vi "TimedLoop-all-inputs-wired.vi"() -> ()   [LabVIEW 2026]
doc: "This VI illustrates how to use the Stop Timed Structure VI to programmatically abort a Timed Loop."
uses:
  <vilib>/Platform/TimedLoop/XDataNode/timing_clust.ctl
  <vilib>/Platform/TimedLoop/XDataNode/nitl_modes.ctl
  <vilib>/Platform/TimedLoop/XDataNode/wakeup.ctl
  <vilib>/platform/TimedLoop/XDataNode/XDataNode.xnode
  <vilib>/Platform/TimedLoop/XDataNode/XDNodeRunTimeDep.lvlib
panel:
  out "Wakeup Reason":string
  in  "Abort Message":string="The Timed Loop was aborted."
  in  "Abort":bool
  out "Current Iteration":i32
  # "Overview: Demonstrates the use of the Stop Timed Structure VI to programmatically abort a Timed Loop.\nRequirements: Windows\nInstructions:\n1. Run the VI.\n2. Click the Abort Timed Loop button. A dialog will indicate that the Timed Loop was programmatically aborted."
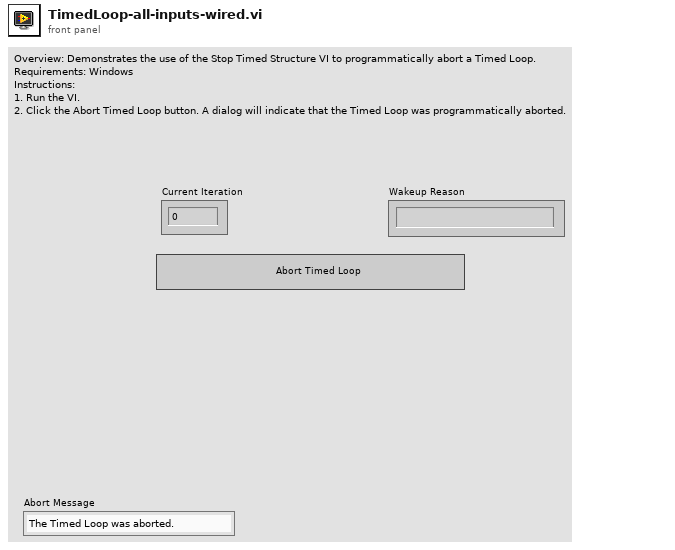
[diagram p1: front panel]
types:
  T1 = typedef "XDNodeRunTimeDep.lvlib/nitl_modes.ctl" = enum32{"No Change", "Process missed periods, maintain original phase", "Discard missed periods, maintain original phase", "Process missed periods, ignore original phase", "Discard missed periods, ignore original phase"}
  T2 = typedef "XDNodeRunTimeDep.lvlib/timing_clust.ctl" = cluster{"Expected End [f-1]":u64, "Actual End [f-1]":u64, "Finished Late? [f-1]":bool, "Expected End [i-1]":u64, "Actual End [i-1]":u64, "Finished Late? [i-1]":bool, "Expected Start [i]":u64, "Actual Start [i]":u64, "Expected Start [f]":u64, "Actual Start [f]":u64, "Source Name":string, "Structure Name":string, "Period":i64, "Deadline":i64, "Offset":i64, "Start":i64, "Priority":i32, "Timeout":i32, "Mode":T1, "Wakeup Reason":T3, "Error":errorcluster, "Source Type":string, "Secondary Source Type":string, "Global End Time":u64, "Global Start Time":u64, "Frame Duration":u64, "Iteration Duration":u64, "Assigned CPU":i32, "I/O Scan Engine Mode":u32}
  T3 = typedef "XDNodeRunTimeDep.lvlib/wakeup.ctl" = enum32{"Normal", "Aborted", "Asynchronous wakeup", "Timing source error", "Timed loop error", "Timeout"}
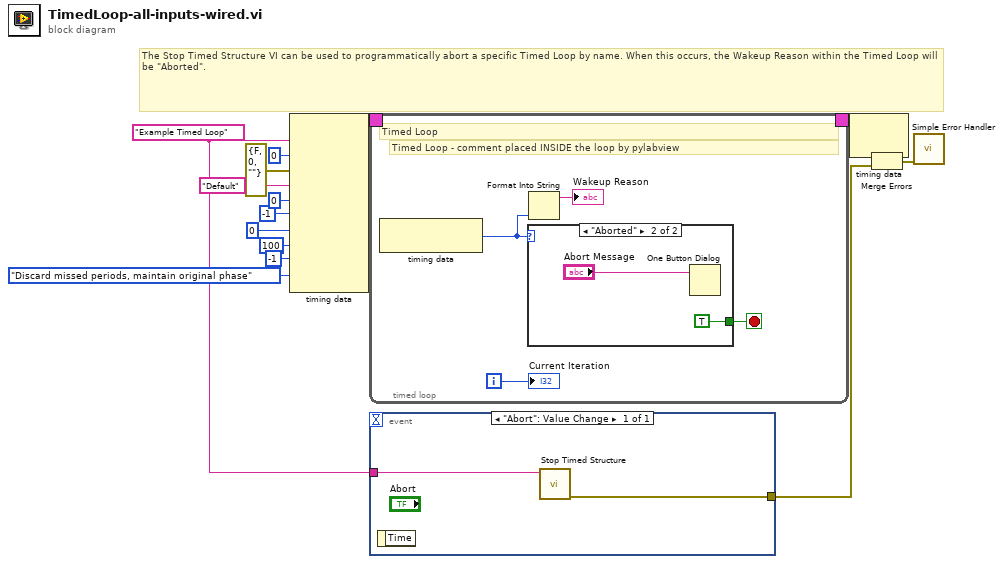
[diagram p0: block diagram]
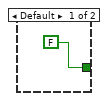
[diagram p2: hidden frame]
diagram:
  w15 = "Example Timed Loop" ("Structure Name")
  # "The Stop Timed Structure VI can be used to programmatically abort a specific Timed Loop by name. When this occurs, the Wakeup Reason within the Timed Loop will be \"Aborted\"."
  n1 = node-c288(w15, 0 ("Processor"), errorcluster {"status"=FALSE, "code"=0, "source"=""} ("Error"), "Default" ("Source Name"), i64 0 ("Period"), i64 -1 ("Deadline"), i64 0 ("Offset"), 100 ("Priority"), -1 ("Timeout"), nitl_modes."Discard missed periods, maintain original phase" ("Mode")) -> (w13:T2)
  n2 = timed-loop {
    timing: w13 -> [_]
    timing-out: [_] -> w14
    i -> [w18]
    stop <- w19 stop-if-true
    # "Timed Loop - comment placed INSIDE the loop by pylabview"
    # "Timed Loop"
    n3 = node-c288() -> (w17:T3)  [unwired: 1 in]
    n4 = case shown="\"Aborted\"" w17 {
      tunnel: [FALSE TRUE] -> w19
      frame Default {
      }
      frame "Aborted" {
        n5 = One Button Dialog(message="Abort Message") -> ()  [unwired: 1 in, 1 out]
      }
    }
    n6 = Format Into String(w17) -> (resulting string=→"Wakeup Reason":string)  [unwired: 3 in, 1 out]
    "Current Iteration" <- w18
  }
  n7 = event shown="[0] \"Abort\": Value Change" {
    selector: _ -> [_]
    dyn-events: _ -> [_]
    timeout: _ -> [_]
    tunnel: w15 -> [w27]
    tunnel: [w26] -> w11
    event "Abort": Value Change {
      n8 = event-data() -> ()  [unwired: 1 in, 1 out]
      n9 = call <vilib>:"Stop Timed Structure.vi"("name"=w27) -> ("error out"=w26:errorcluster)  [unwired: 10 in]
    }
  }
  n10 = node-c288(w14) -> (w12:errorcluster)
  n11 = Merge Errors(w12, w11) -> (w10:errorcluster)
  n12 = call <vilib>:"Simple Error Handler.vi"("error in (no error)"=w10) -> ()  [unwired: 4 in, 5 out]
